vi "Replace Item Property.vi"(8 "error in (no error)":errorcluster, 9 "Replace Value":string, 10 "Replace Column":T1, 11 "Item in":refnum<class "Item.lvclass">) -> (0 "error out":errorcluster, 3 "Item out":refnum<class "Item.lvclass">)   [LabVIEW 2020, in "VI Properties Editor.lvlib" / "Item.lvclass"]
doc: "Replaces the value of the property identified by <B>Replace Column</B> with <B>Replace Value</B>."
uses:
  Item.lvclass
  CTLs/Replace Column.ctl
  VI Properties Editor.lvlib
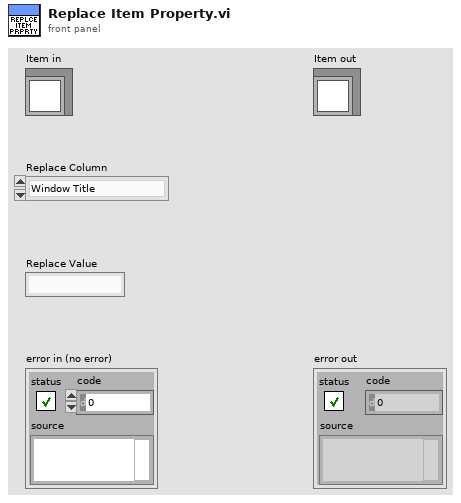
[diagram p1: front panel]
types:
  T1 = typedef "VI Properties Editor.lvlib/Replace Column.ctl" = enum16{"Window Title", "Description", "Help Path", "Help Tag", "Custom Title?", "Help URL", "Help Type", "Control Label", "Control Caption", "Control Description", "Control Tip Strip"}
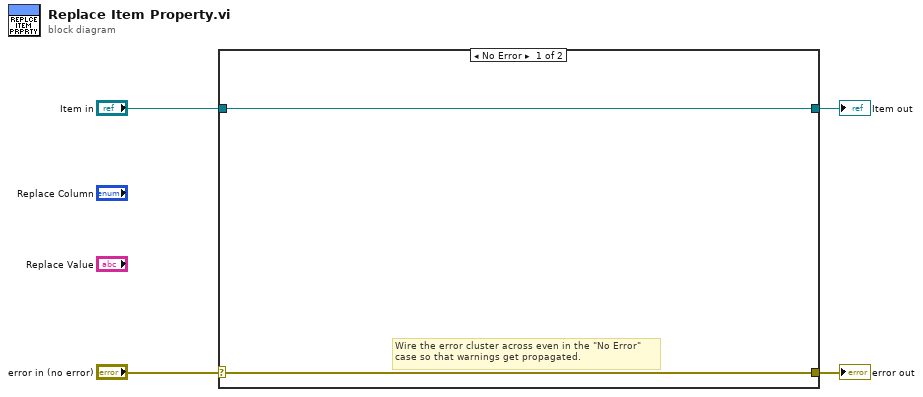
[diagram p0: block diagram]
diagram:
  n1 = case shown="No Error" "error in (no error)" {
    selector: "error in (no error)" -> [w5 w8]
    tunnel: [w5 w8] -> w3
    tunnel: [w6 w7] -> w1
    tunnel: "Item in" -> [w6 w7]
    frame No Error {
      # "Wire the error cluster across even in the \"No Error\"\ncase so that warnings get propagated."
    }
    frame Error {
    }
  }
  "error out" <- w3
  "Item out" <- w1
